vi "PID Align Correction.vi"(0 "Robot Velocities":T4, 1 "Zero V":bool, 2 "Expected Position":cluster{"x":dbl, "y":dbl, "th":dbl}, 3 "Final Position":cluster{"x":dbl, "y":dbl, "th":dbl}, 4 "Path Finished?":bool=TRUE) -> (5 "Final velocity":T4, 6 "PID happy":bool=TRUE)   [LabVIEW 2025]
uses:
  swerve-template/Type Definitions/Data/Robot Velocities.ctl
  Implementation/Tune Auto Pickup PID.ctl
  <vilib>/Rock Robotics/Network Tables/NT Read Numeric Array.vi
panel:
  out "Error":cluster{"X":dbl, "Y":dbl, "Theta":dbl}={"X"=0.009854650689625544, "Y"=0.14740072303684304, "Theta"=1.1601458496305803}
  in  "Theta Booleans":cluster{"PID Off?":bool, "Invert value":bool}
  in  "Y Booleans":cluster{"PID Off?":bool, "Invert value":bool}={"PID Off?"=FALSE, "Invert value"=TRUE}
  in  "X Booleans":cluster{"PID Off?":bool, "Invert value":bool}
  out "Debug Graph":cluster{"sine wave":dbl, "Theta":dbl}(graph)={"sine wave"=-11.72322778883767, "Theta"=-17.14660154582522}
  in  "Debug Input":T2={"amplitude \n(ft or degrees)"=20.0, "frequency (sec)"=0.1, "Tune Align PID"=enum."Not Enabled"} {"frequency (sec)" format="%0.2f"; "amplitude \n(ft or degrees)" format="%0.2f"}
  in  "PID Deadband":cluster{"x":dbl, "y":dbl, "th":dbl}={"x"=0.25, "y"=0.25, "th"=10.0}
  in  "PID inputs rotational":T3={"output range"={"high"=80.0, "low"=-80.0}, "PID gains"={"proportional gain (Kp)"=2.0, "integral time (Ki)"=0.0, "derivative time (Kd)"=0.0}} {"output range"."low" format="%.2f"; "output range"."high" format="%.2f"; "PID gains"."derivative time (Kd)" format="%.6f"; "PID gains"."integral time (Ki)" format="%.6f"; "PID gains"."proportional gain (Kp)" format="%.6f"}
  in  "PID inputs translational":T3={"output range"={"high"=8.0, "low"=-8.0}, "PID gains"={"proportional gain (Kp)"=1.0, "integral time (Ki)"=0.0, "derivative time (Kd)"=0.0}} {"output range"."low" format="%.2f"; "output range"."high" format="%.2f"; "PID gains"."derivative time (Kd)" format="%.6f"; "PID gains"."integral time (Ki)" format="%.6f"; "PID gains"."proportional gain (Kp)" format="%.6f"}
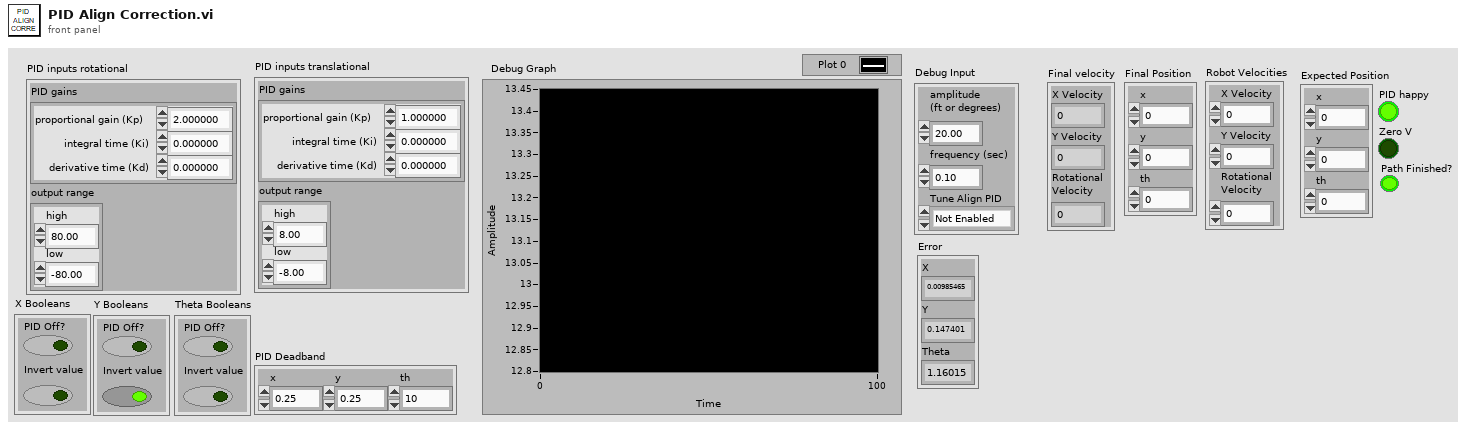
[diagram p1: front panel]
types:
  T1 = typedef "Tune Auto Pickup PID.ctl" = enum16{"Not Enabled", "X Axis", "Y Axis", "Theta"}
  T2 = cluster{"amplitude \n(ft or degrees)":dbl, "frequency (sec)":dbl, "Tune Align PID":T1}
  T3 = cluster{"output range":cluster{"high":dbl, "low":dbl}, "PID gains":cluster{"proportional gain (Kp)":dbl, "integral time (Ki)":dbl, "derivative time (Kd)":dbl}}
  T4 = typedef "Robot Velocities.ctl" = cluster{"X Velocity":dbl, "Y Velocity":dbl, "Rotational \nVelocity":dbl}
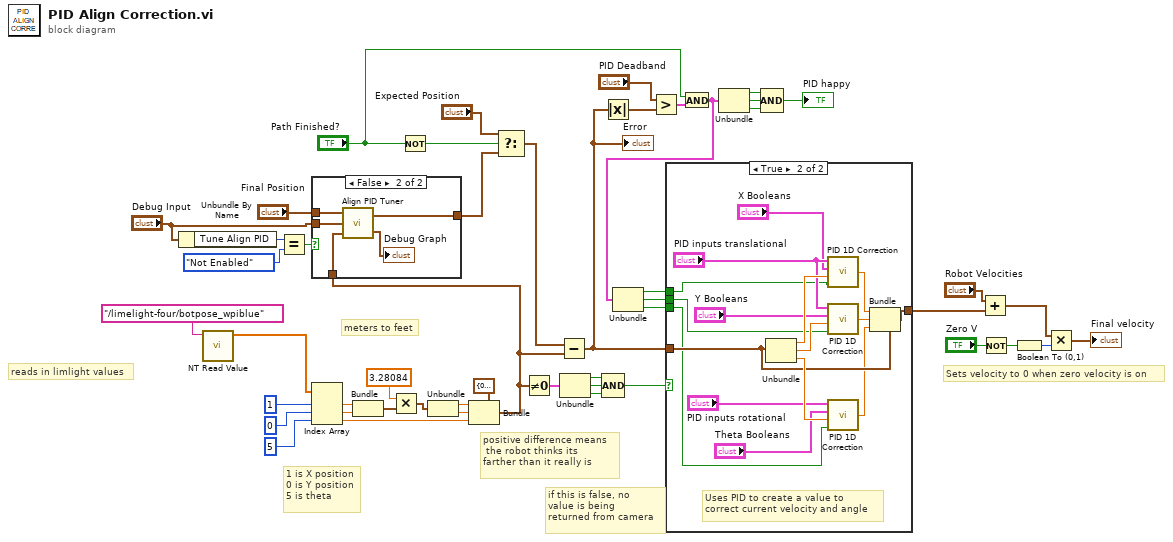
[diagram p0: block diagram]
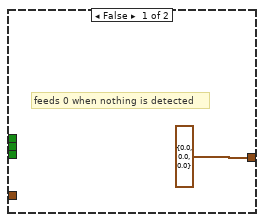
[diagram p3: hidden frame]
diagram:
  # "meters to feet"
  # "reads in limlight values"
  # "1 is X position\n0 is Y position\n5 is theta"
  # "if this is false, no \nvalue is being \nreturned from camera"
  # "positive difference means\n the robot thinks its\nfarther than it really is"
  # "Sets velocity to 0 when zero velocity is on"
  n1 = Unbundle By Name("Debug Input") -> ("Tune Align PID"=w29:T1)
  n2 = call-poly <vilib>:"NT Read Value.vi"("name"="/limelight-four/botpose_wpiblue") -> ("value"=w19:dbl[])  [unwired: 8 in, 2 out]
  n3 = Equal?(x=w29, y=Tune_Auto_Pickup_PID."Not Enabled") -> (x = y?=w30:bool)
  n4 = Index Array(array=w19, index #1=1 ("index"), index #2=0 ("index"), index #3=5 ("index")) -> (element #1=w14:dbl, element #2=w13:dbl, element #3=w22:dbl)
  n5 = Bundle("Numeric"=w14, "Numeric"=w13) -> (w18:cluster{"Numeric":dbl, "Numeric":dbl})  [unwired: 1 in]
  n6 = Multiply(x=3.28084, y=w18) -> (x*y=w17:cluster{"Numeric":dbl, "Numeric":dbl})
  n7 = Not(x="Path Finished?") -> (.not. x?=w11:bool)
  n8 = Unbundle(w17) -> ("Numeric"=w16:dbl, "Numeric"=w15:dbl)
  n9 = Bundle(cluster=cluster{"X":dbl, "Y":dbl, "Theta":dbl} {"X"=0.0, "Y"=0.0, "Theta"=0.0}, "X"=w16, "Y"=w15, "Theta"=w22) -> (w9:cluster{"X":dbl, "Y":dbl, "Theta":dbl})
  n10 = case shown="False" w30 {
    tunnel: "Debug Input" -> [_ w52]
    tunnel: "Final Position" -> [w50 w53]
    tunnel: [w50 w54] -> w26
    tunnel: w9 -> [_ w51]
    frame True {
    }
    frame False {
      n11 = call "Align PID Tuner.vi"("Current Position"=w51, "Debug Input"=w52, "Final Position"=w53) -> ("Graph Data"=→"Debug Graph":cluster{"Error":dbl, "Exppected":dbl}, "Sine Corrected Positions"=w54:cluster{"X":dbl, "Y":dbl, "Theta":dbl})
    }
  }
  n12 = Select(t="Expected Position", s=w11, f=w26) -> (s? t:f=w42:cluster{"X":dbl, "Y":dbl, "Theta":dbl})
  n13 = Not Equal To 0?(x=w9) -> (x != 0?=w40:cluster{"X":bool, "Y":bool, "Theta":bool})
  n14 = Subtract(x=w42, y=w9) -> (x-y=w8:cluster{"X":dbl, "Y":dbl, "Theta":dbl})
  "Error" <- w8
  n15 = Unbundle(w40) -> ("X"=w39:bool, "Y"=w38:bool, "Theta"=w37:bool)
  n16 = Compound Arithmetic op=AND(w39, w38, w37) -> (w41:bool)
  n17 = Absolute Value(x=w8) -> (abs(x)=w34:cluster{"X":dbl, "Y":dbl, "Theta":dbl})
  n18 = Greater?(x="PID Deadband", y=w34) -> (0:w7:cluster{bool, bool, bool})
  n19 = And(x="Path Finished?", y=w7) -> (x .and. y?=w1:cluster{bool, bool, bool})
  n20 = Unbundle(w1) -> (w2:bool, w3:bool, w4:bool)
  n21 = case shown="True" w41 {
    tunnel: [cluster{"x":dbl, "y":dbl, "th":dbl} {"x"=0.0, "y"=0.0, "th"=0.0} w69] -> w47
    tunnel: w8 -> [_ w68]
    tunnel: w4 -> [_ w59]
    tunnel: w3 -> [_ w58]
    tunnel: w2 -> [_ w57]
    frame False {
      # "feeds 0 when nothing is detected"
    }
    frame True {
      # "Uses PID to create a value to\ncorrect current velocity and angle"
      n22 = Unbundle(w68) -> ("X"=w71:dbl, "Y"=w72:dbl, "Theta"=w70:dbl)
      n23 = call "PID 1D Correction.vi"("In Range?"=w57, "Distance off"=w71, "PID Booleans"="X Booleans", "PID inputs"="PID inputs translational") -> ("Correction"=w67:dbl)
      n24 = call "PID 1D Correction.vi"("In Range?"=w58, "Distance off"=w72, "PID Booleans"="Y Booleans", "PID inputs"="PID inputs translational") -> ("Correction"=w66:dbl)
      n25 = call "PID 1D Correction.vi"("In Range?"=w59, "Distance off"=w70, "PID Booleans"="Theta Booleans", "PID inputs"="PID inputs rotational") -> ("Correction"=w65:dbl)
      n26 = Bundle(cluster=w68, "X"=w67, "Y"=w66, "Theta"=w65) -> (w69:cluster{"X":dbl, "Y":dbl, "Theta":dbl})
    }
  }
  n27 = Unbundle(w1) -> (w32:bool, w36:bool, w35:bool)
  n28 = Compound Arithmetic op=AND(w32, w36, w35) -> (→"PID happy":bool)
  n29 = Add(x="Robot Velocities", y=w47) -> (x+y=w44:T4)
  n30 = Not(x="Zero V") -> (.not. x?=w48:bool)
  n31 = Boolean To (0,1)(Boolean=w48) -> (0, 1=w45:i16)
  n32 = Multiply(x=w44, y=w45) -> (x*y=→"Final velocity":T4)
